vi "Configure.vi"(6 "Impedancia":enum16{"50", "600", "HiZ"}(ring), 8 "error in (no error)":errorcluster, 9 "Frequency (Hz)":dbl=10.0, 10 "Amplitude (Vrms)":dbl=5.0, 11 "VISA resource name":refnum<visa-resource-name>) -> (0 "error out":errorcluster, 3 "VISA resource name out":refnum<visa-resource-name>)   [LabVIEW 2019, in "DS360.lvlib"]
uses:
  DS360.lvlib
panel:
  out "resulting string":string
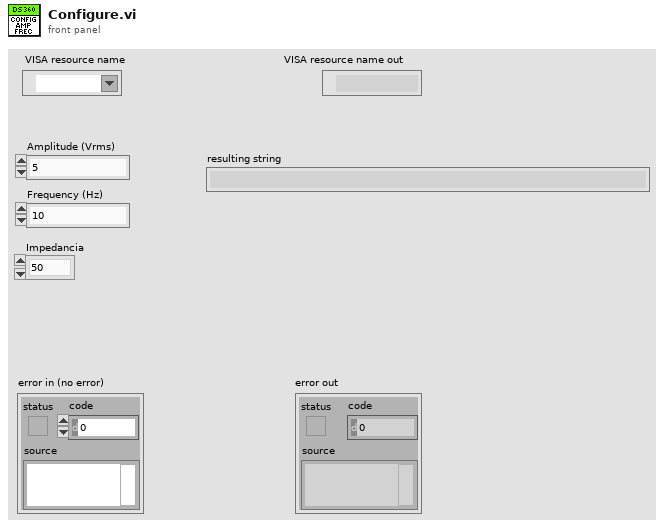
[diagram p1: front panel]
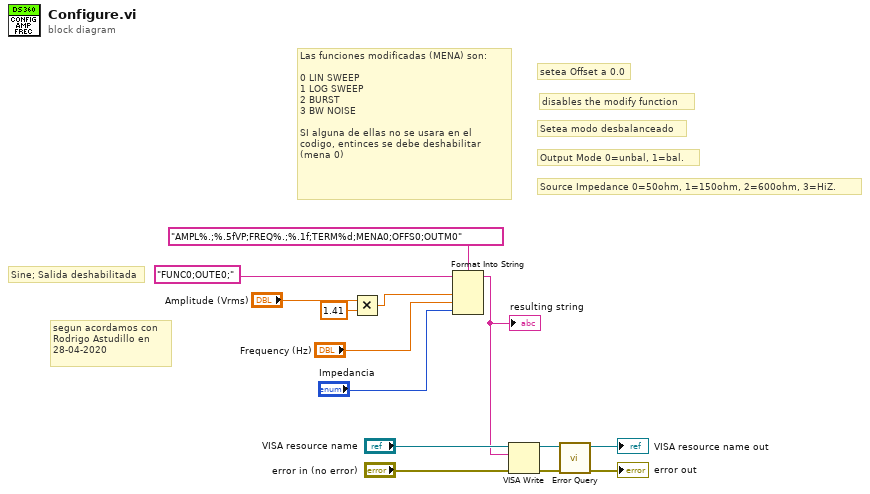
[diagram p0: block diagram]
diagram:
  # "disables the modify function"
  # "Source Impedance 0=50ohm, 1=150ohm, 2=600ohm, 3=HiZ."
  # "Output Mode 0=unbal, 1=bal."
  # "Setea modo desbalanceado"
  # "setea Offset a 0.0"
  # "Las funciones modificadas (MENA) son:\n\n0 LIN SWEEP\n1 LOG SWEEP\n2 BURST\n3 BW NOISE\n\nSI alguna de ellas no se usara en el\ncodigo, entinces se debe deshabilitar\n(mena 0)"
  # "segun acordamos con\nRodrigo Astudillo en\n28-04-2020"
  # "Sine; Salida deshabilitada"
  n1 = Multiply(x="Amplitude (Vrms)", y=1.41) -> (x*y=w3:dbl)
  n2 = Format Into String(format string="AMPL%.;%.5fVP;FREQ%.;%.1f;TERM%d;MENA0;OFFS0;OUTM0", initial string="FUNC0;OUTE0;" ("string (\"\")"), w3, "Frequency (Hz)", "Impedancia") -> (resulting string=w1:string)  [unwired: 1 in, 1 out]
  "resulting string" <- w1
  n3 = VISA Write(VISA resource name="VISA resource name", write buffer=w1, error in (no error)="error in (no error)") -> (VISA resource name out=w10:refnum<visa-resource-name>, error out=w9:errorcluster)  [unwired: 1 out]
  n4 = call "Error Query.vi"("error in (no error)"=w9, "VISA resource name"=w10) -> ("error out"=→"error out":errorcluster, "VISA resource name out"=→"VISA resource name out":refnum<visa-resource-name>)  [unwired: 6 in, 2 out]
